vi "PCO_PlayImagesFromSegmentHDSDI.vi"(0 "ph":u64, 1 "wSpeed":u16, 2 "dwRangeHigh":u32, 5 "wSegment":u16, 7 "wInterface":u16, 9 "wMode":u16(ring) items=["stop"=0, "play fast forward, no replay"=1, "play fast backward, no replay"=2, "play slow forward, no replay"=3, "play slow backward, no replay"=4, "play fast forward, replay"=257, "play fast backward, replay"=258, "play slow forward, replay"=259, "play slow backward, replay"=260], 11 "error in (no error)":errorcluster {"code" format="%x"}, 12 "dwRangeLow":u32, 13 "dwStartPos":u32) -> (4 "ph out":u64, 6 "ErrorMessage":i32 format="%x", 15 "error out":errorcluster {"code" format="%x"})   [LabVIEW 2019, in "SDK.lvlib" / "SpecialCommandsDimax_HDSDI.lvlib"]
doc: "<b>Description:</b>\nThis function does setup the image output on the HD-SDI interface.\nIt is used to stream the recorded images from the camera internal memory (CamRAM) to the HD-SDI interface. The HD-SDI interface is an output only interface, therefore it does not request images, but it has to be supplied with a continuous data stream.\nThis function can only be used, if PCO_SetStorageMode is set to [recorder] and recording to the camera RAM segment is stopped.\nIf PCO_PlayImagesFromSegmentHDSDI is called, the sequence is started and the function returns immediately. Streaming time for the entire recorded sequence may take seconds or up to minutes depending on the choosen parameters.\nThe play speed is defined by the wSpeed parameter together with the wMode parameter:\n• Fast forward: The play position is increased by wSpeed, so (wSpeed-1) images are leaped\n• Fast rewind: The play position is decreased by wSpeed, so (wSpeed-1) images are leaped\n• Slow forward: The current image is sent wSpeed times before the position is increased\n• Slow rewind: The current image is sent wSpeed times before the position is decreased\nWith the play command parameters (e.g. wSpeed) can also be changed while a play is active. The parameters will be changed immediately. It is possible to change parameters like play speed or play direction without changing the current position by setting Start No. to -1 (asDWORD 0xFFFFFFFF ).\n\n<b>Supported camera type:</b>\npco.dimax with HD-SDI interface\n\n<b>Descriptor dependency:</b>\nNone"
uses:
  SpecialCommandsDimax_HDSDI.lvlib
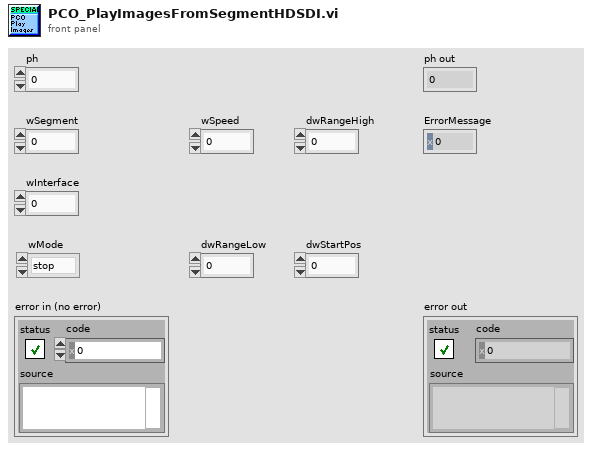
[diagram p1: front panel]
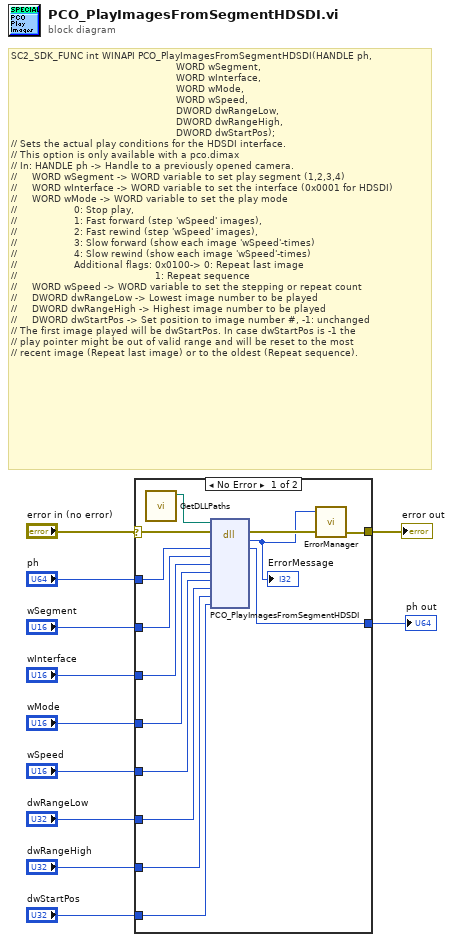
[diagram p0: block diagram]
diagram:
  # "SC2_SDK_FUNC int WINAPI PCO_PlayImagesFromSegmentHDSDI(HANDLE ph,\n                                                       WORD wSegment,\n                                                       WORD wInterface,\n                                                       WORD wMode,\n                                                       WORD wSpeed,\n                                                       DWORD dwRangeLow,\n                                                       DWORD dwRangeHigh,\n                                                       DWORD dwStartPos);\n// Sets the actual play conditions for the HDSDI interface.\n// This option is only available with a pco.dimax\n// In: HANDLE ph -> Handle to a previously opened camera.\n//     WORD wSegment -> WORD variable to set play segment (1,2,3,4)\n//     WORD wInterface -> WORD variable to set the interface (0x0001 for HDSDI)\n//     WORD wMode -> WORD variable to set the play mode\n//                   0: Stop play,\n//                   1: Fast forward (step 'wSpeed' images),\n//                   2: Fast rewind (step 'wSpeed' images), \n//                   3: Slow forward (show each image 'wSpeed'-times)\n//                   4: Slow rewind (show each image 'wSpeed'-times)\n//                   Additional flags: 0x0100-> 0: Repeat last image\n//                                              1: Repeat sequence\n//     WORD wSpeed -> WORD variable to set the stepping or repeat count\n//     DWORD dwRangeLow -> Lowest image number to be played\n//     DWORD dwRangeHigh -> Highest image number to be played\n//     DWORD dwStartPos -> Set position to image number #, -1: unchanged\n// The first image played will be dwStartPos. In case dwStartPos is -1 the\n// play pointer might be out of valid range and will be reset to the most\n// recent image (Repeat last image) or to the oldest (Repeat sequence)."
  n1 = case shown="No Error" "error in (no error)" {
    selector: "error in (no error)" -> [w16 w27]
    tunnel: "ph" -> [w25 w26]
    tunnel: [w24 w26] -> w10
    tunnel: "wSegment" -> [w23 _]
    tunnel: "wInterface" -> [w22 _]
    tunnel: "wMode" -> [w21 _]
    tunnel: "wSpeed" -> [w20 _]
    tunnel: "dwRangeLow" -> [w19 _]
    tunnel: "dwRangeHigh" -> [w18 _]
    tunnel: "dwStartPos" -> [w17 _]
    tunnel: [w15 w27] -> w2
    frame No Error {
      n2 = call "GetDLLPaths.vi"() -> ("SC2_Cam_Path"=w12:path)  [unwired: 9 in, 2 out]
      n3 = dll-call lib="?" fn="PCO_PlayImagesFromSegmentHDSDI"(path in=w12, error in=w16, "ph"=w25, "wSegment"=w23, "wInterface"=w22, "wMode"=w21, "wSpeed"=w20, "dwRangeLow"=w19, "dwRangeHigh"=w18, "dwStartPos"=w17) -> (error out=w14:errorcluster, "return type"=w13:i32, "ph"=w24:u64)  [unwired: 8 in, 1 out]
      "ErrorMessage" <- w13
      n4 = call "ErrorManager.vi"("error in (no error)"=w14, "error code"=w13) -> ("error out"=w15:errorcluster)  [unwired: 3 in]
    }
    frame Error {
    }
  }
  "ph out" <- w10
  "error out" <- w2
